vi "Init TCP (Direct).vi"(7 "Error Checking (Full)":T1=enum."Full", 8 "error in (no error)":errorcluster, 11 "VISA resource name":refnum<visa-resource-name>) -> (0 "error out":errorcluster, 3 "VisaComms out":refnum<class "VisaComms.lvclass">)   [LabVIEW 2024, in "CTI.lvlib" / "VisaComms.lvclass"]
uses:
  VisaComms.lvclass
  Error Reporting.ctl
  <vilib>/Instr/_visa.llb/VISA Open Access Mode.ctl
  VisaComms.lvclass/VisaComms.ctl
  CTI.lvlib
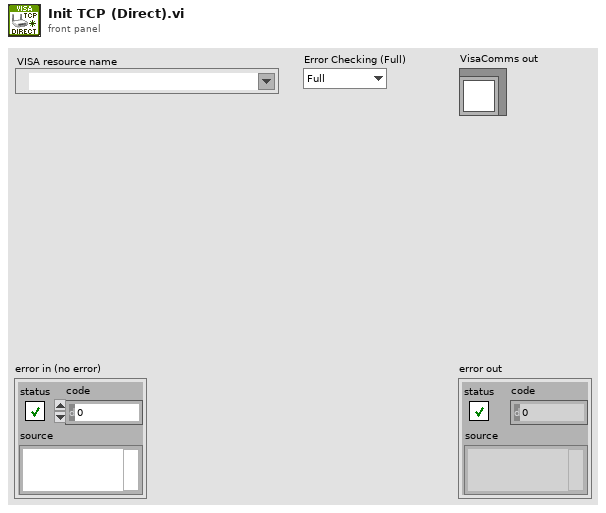
[diagram p1: front panel]
types:
  T1 = typedef "CTI.lvlib/Error Reporting.ctl" = enum16{"Minimal", "Moderate", "Full"}
  T2 = typedef "VISA Open Access Mode.ctl" = u32
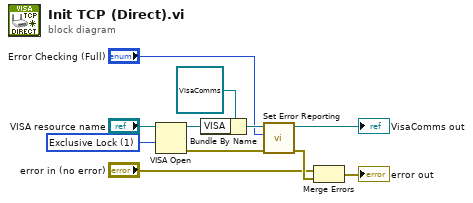
[diagram p0: block diagram]
diagram:
  w9 = T2 1 items=["VISA Defaults"=0, "Exclusive Lock"=1, "Load Configured Settings"=4] ("Access Mode")
  n1 = VISA Open(access mode=w9, VISA resource name="VISA resource name") -> (VISA resource name=w10:refnum<visa-resource-name>, error out=w7:errorcluster)  [unwired: 3 in]
  n2 = Bundle By Name(cluster=refnum<class "VisaComms.lvclass"> refnum ("CTI.lvlib:VisaComms.lvclass"), "VISA"=w10) -> (w8:refnum<class "VisaComms.lvclass">)
  n3 = call-dynamic "Set Error Reporting.vi"("error in (no error)"=w7, "Error Reporting"="Error Checking (Full)", "VisaComms in"=w8) -> ("error out"=w6:errorcluster, "VisaComms out"=→"VisaComms out":refnum<class "VisaComms.lvclass">)  [unwired: 7 in]
  n4 = Merge Errors("error in (no error)", w6) -> (→"error out":errorcluster)
